vi "test_read-nmea-data2.vi"() -> ()   [LabVIEW 2019] (continued)
\n15:14:24.49\tF9P\t$GLGSV,2,1,08,69,10,031,37,70,70,037,25,71,54,207,25,72,05,210,,1*7E\n\t\n15:14:24.51\tF9P\t$GLGSV,2,2,08,77,01,325,,84,19,123,19,85,70,070,27,86,37,330,,1*7B\n\t\n15:14:24.53\tF9P\t$GLGSV,2,1,08,69,10,031,26,70,70,037,,71,54,207,16,72,05,210,,3*7B\n\t\n15:14:24.55\tF9P\t$GLGSV,2,2,08,77,01,325,,84,19,123,24,85,70,070,22,86,37,330,,3*72\n\t\n15:14:24.57\tF9P\t$GAGSV,2,1,08,02,08,296,11,04,67,115,26,09,33,193,24,11,72,001,24,7*7D\n\t\n15:14:24.59\tF9P\t$GAGSV,2,2,08,12,39,103,31,19,25,045,28,25,08,248,,36,27,309,18,7*74\n\t\n15:14:24.61\tF9P\t$GAGSV,2,1,08,02,08,296,,04,67,115,,09,33,193,,11,72,001,23,2*7D\n\t\n15:14:24.63\tF9P\t$GAGSV,2,2,08,12,39,103,27,19,25,045,,25,08,248,,36,27,309,,2*75\n\t\n15:14:24.65\tF9P\t$GBGSV,2,1,05,07,,,31,11,48,133,30,14,87,101,26,28,,,27,1*7A\n\t\n15:14:24.67\tF9P\t$GBGSV,2,2,05,33,62,220,24,1*41\n\t\n15:14:24.69\tF9P\t$GBGSV,1,1,03,11,48,133,31,14,87,101,28,33,62,220,,3*4C\n\t\n15:14:24.71\tF9P\t$GNGLL,3723.59802,N,12656.97828,E,061426.00,A,A*79\n\t\n15:14:24.73\tF9P\t\t\n15:14:24.75\tF9P\t\t\n15:14:24.77\tF9P\t\t\n15:14:24.79\tF9P\t\t\n15:14:24.81\tF9P\t\t\n15:14:24.83\tF9P\t\t\n15:14:24.85\tF9P\t\t\n15:14:24.87\tF9P\t\t\n15:14:24.89\tF9P\t\t\n15:14:24.91\tF9P\t\t\n15:14:24.93\tF9P\t\t\n15:14:24.95\tF9P\t\t\n15:14:24.97\tF9P\t\t\n15:14:24.99\tF9P\t\t\n15:14:25.01\tF9P\t\t\n15:14:25.03\tF9P\t\t\n15:14:25.05\tF9P\t\t\n15:14:25.07\tF9P\t\t\n15:14:25.09\tF9P\t\t\n15:14:25.11\tF9P\t\t\n15:14:25.13\tF9P\t\t\n15:14:25.15\tF9P\t\t\n15:14:25.17\tF9P\t\t\n15:14:25.19\tF9P\t\t\n15:14:25.21\tF9P\t\t\n15:14:25.23\tF9P\t$GNRMC,061427.00,A,3723.59868,N,12656.97826,E,2.049,344.09,25072\t\n15:14:25.25\tF9P\t0,,,A,V*00\n\t\n15:14:25.27\tF9P\t$GNVTG,344.09,T,,M,2.049,N,3.795,K,A*2E\n\t\n15:14:25.29\tF9P\t$GNGGA,061427.00,3723.59868,N,12656.97826,E,1,12,0.66,44.3,M,18.5,M,,*73\n\t\n15:14:25.31\tF9P\t$GNGSA,A,3,12,06,19,05,17,09,04,02,,,,,1.17,0.66,0.97,1*09\n\t\n15:14:25.33\tF9P\t$GNGSA,A,3,85,70,71,84,,,,,,,,,1.17,0.66,0.97,2*0B\n\t\n15:14:25.35\tF9P\t$GNGSA,A,3,36,19,11,04,09,12,,,,,,,1.17,0.66,0.97,3*09\n\t\n15:14:25.37\tF9P\t$GNGSA,A,3,14,11,33,,,,,,,,,,1.17,0.66,0.97,4*08\n\t\n15:14:25.39\tF9P\t$GPGSV,3,1,09,02,55,320,27,04,17,043,34,05,38,248,34,06,64,050,32,1*6C\n\t\n15:14:25.41\tF9P\t$GPGSV,3,2,09,09,44,073,31,12,23,276,30,17,32,154,27,19,51,157,30,1*6F\n\t\n15:14:25.43\tF9P\t$GPGSV,3,3,09,25,12,306,20,1*5E\n\t\n15:14:25.45\tF9P\t$GPGSV,3,1,09,02,55,320,,04,17,043,22,05,38,248,21,06,64,050,25,6*6B\n\t\n15:14:25.47\tF9P\t$GPGSV,3,2,09,09,44,073,25,12,23,276,14,17,32,154,23,19,51,157,,6*6C\n\t\n15:14:25.49\tF9P\t$GPGSV,3,3,09,25,12,306,,6*5B\n\t\n15:14:25.51\tF9P\t$GLGSV,2,1,08,69,10,031,35,70,70,037,24,71,54,207,25,72,05,210,,1*7D\n\t\n15:14:25.53\tF9P\t$GLGSV,2,2,08,77,01,325,,84,19,123,20,85,70,070,32,86,37,330,,1*75\n\t\n15:14:25.55\tF9P\t$GLGSV,2,1,08,69,10,031,26,70,70,037,,71,54,207,14,72,05,210,,3*79\n\t\n15:14:25.57\tF9P\t$GLGSV,2,2,08,77,01,325,,84,19,123,24,85,70,070,22,86,37,330,,3*72\n\t\n15:14:25.59\tF9P\t$GAGSV,2,1,08,02,08,296,08,04,67,115,25,09,33,193,24,11,72,001,25,7*77\n\t\n15:14:25.61\tF9P\t$GAGSV,2,2,08,12,39,103,27,19,25,045,29,25,08,248,,36,27,309,14,7*7E\n\t\n15:14:25.63\tF9P\t$GAGSV,2,1,08,02,08,296,,04,67,115,,09,33,193,,11,72,001,24,2*7A\n\t\n15:14:25.65\tF9P\t$GAGSV,2,2,08,12,39,103,25,19,25,045,,25,08,248,,36,27,309,,2*77\n\t\n15:14:25.67\tF9P\t$GBGSV,2,1,06,07,,,31,11,48,133,33,14,87,101,26,28,,,27,1*7A\n\t\n15:14:25.69\tF9P\t$GBGSV,2,2,06,33,62,220,26,34,,,43,1*40\n\t\n15:14:25.71\tF9P\t$GBGSV,1,1,03,11,48,133,30,14,87,101,,33,62,220,,3*47\n\t\n15:14:25.73\tF9P\t$GNGLL,3723.59868,N,12656.97826,E,061427.00,A,A*7A\n\t\n15:14:25.75\tF9P\t\t\n15:14:25.77\tF9P\t\t\n15:14:25.79\tF9P\t\t\n15:14:25.81\tF9P\t\t\n15:14:25.83\tF9P\t\t\n15:14:25.85\tF9P\t\t\n15:14:25.87\tF9P\t\t\n15:14:25.89\tF9P\t\t\n15:14:25.91\tF9P\t\t\n15:14:25.93\tF9P\t\t\n15:14:25.95\tF9P\t\t\n15:14:25.97\tF9P\t\t\n15:14:25.99\tF9P\t\t\n15:14:26.01\tF9P\t\t\n15:14:26.03\tF9P\t\t\n15:14:26.05\tF9P\t\t\n15:14:26.07\tF9P\t\t\n15:14:26.09\tF9P\t\t\n15:14:26.11\tF9P\t\t\n15:14:26.13\tF9P\t\t\n15:14:26.15\tF9P\t\t\n15:14:26.17\tF9P\t\t\n15:14:26.19\tF9P\t\t\n15:14:26.21\tF9P\t\t\n15:14:26.23\tF9P\t$GNRMC,061428.00,A,3723.59932,N,12656.97803,E,1.624,347.59,250720,,,A,V*0E\n\t\n15:14:26.25\tF9P\t$GNVTG,347.59,T,,M,1.624,N,3.007,K,A*2A\n\t\n15:14:26.27\tF9P\t$GNGGA,061428.00,3723.59932,N,12656.97803,E,1,12,0.71,44.3,M,18.5,M,,*73\n\t\n15:14:26.29\tF9P\t$GNGSA,A,3,12,06,19,05,17,09,04,02,,,,,1.23,0.71,1.01,1*06\n\t\n15:14:26.31\tF9P\t$GNGSA,A,3,85,70,71,84,,,,,,,,,1.23,0.71,1.01,2*04\n\t\n15:14:26.33\tF9P\t$GNGSA,A,3,36,19,11,04,09,12,,,,,,,1.23,0.71,1.01,3*06\n\t\n15:14:26.35\tF9P\t$GNGSA,A,3,14,11,33,,,,,,,,,,1.23,0.71,1.01,4*07\n\t\n15:14:26.37\tF9P\t$GPGSV,3,1,09,02,55,320,28,04,17,043,30,05,38,248,37,06,64,050,27,1*60\n\t\n15:14:26.39\tF9P\t$GPGSV,3,2,09,09,44,073,32,12,23,276,22,17,32,154,36,19,51,157,34,1*6B\n\t\n15:14:26.41\tF9P\t$GPGSV,3,3,09,25,12,306,21,1*5F\n\t\n15:14:26.43\tF9P\t$GPGSV,3,1,09,02,55,320,,04,17,043,22,05,38,248,20,06,64,050,26,6*69\n\t\n15:14:26.45\tF9P\t$GPGSV,3,2,09,09,44,073,26,12,23,276,15,17,32,154,23,19,51,157,,6*6E\n\t\n15:14:26.47\tF9P\t$GPGSV,3,3,09,25,12,306,,6*5B\n\t\n15:14:26.49\tF9P\t$GLGSV,2,1,08,69,10,031,28,70,70,037,23,71,54,207,24,72,05,210,,1*77\n\t\n15:14:26.51\tF9P\t$GLGSV,2,2,08,77,01,325,,84,19,123,20,85,70,070,33,86,37,330,,1*74\n\t\n15:14:26.53\tF9P\t$GLGSV,2,1,08,69,10,031,25,70,70,037,,71,54,207,15,72,05,210,,3*7B\n\t\n15:14:26.55\tF9P\t$GLGSV,2,2,08,77,01,325,,84,19,123,22,85,70,070,22,86,37,330,,3*74\n\t\n15:14:26.57\tF9P\t$GAGSV,2,1,08,02,08,296,10,04,67,115,31,09,33,193,24,11,72,001,25,7*7B\n\t\n15:14:26.59\tF9P\t$GAGSV,2,2,08,12,39,103,24,19,25,045,28,25,08,248,,36,27,309,12,7*7A\n\t\n15:14:26.61\tF9P\t$GAGSV,2,1,08,02,08,296,,04,67,115,,09,33,193,,11,72,001,,2*7C\n\t\n15:14:26.63\tF9P\t$GAGSV,2,2,08,12,39,103,23,19,25,045,,25,08,248,,36,27,309,,2*71\n\t\n15:14:26.65\tF9P\t$GBGSV,2,1,06,07,,,36,11,48,133,31,14,87,101,26,28,,,26,1*7E\n\t\n15:14:26.67\tF9P\t$GBGSV,2,2,06,33,62,220,42,34,,,40,1*41\n\t\n15:14:26.69\tF9P\t$GBGSV,1,1,03,11,48,133,,14,87,101,,33,62,220,,3*44\n\t\n15:14:26.71\tF9P\t$GNGLL,3723.59932,N,12656.97803,E,061428.00,A,A*7C\n\t\n15:14:26.73\tF9P\t\t\n15:14:26.75\tF9P\t\t\n15:14:26.77\tF9P\t\t\n15:14:26.79\tF9P\t\t\n15:14:26.81\tF9P\t\t\n15:14:26.83\tF9P\t\t\n15:14:26.85\tF9P\t\t\n15:14:26.87\tF9P\t\t\n15:14:26.89\tF9P\t\t\n15:14:26.91\tF9P\t\t\n15:14:26.93\tF9P\t\t\n15:14:26.95\tF9P\t\t\n15:14:26.97\tF9P\t\t\n15:14:26.99\tF9P\t\t\n15:14:27.01\tF9P\t\t\n15:14:27.03\tF9P\t\t\n15:14:27.05\tF9P\t\t\n15:14:27.07\tF9P\t\t\n15:14:27.09\tF9P\t\t\n15:14:27.11\tF9P\t\t\n15:14:27.13\tF9P\t\t\n15:14:27.15\tF9P\t\t\n15:14:27.17\tF9P\t\t\n15:14:27.19\tF9P\t\t\n15:14:27.21\tF9P\t\t\n15:14:27.23\tF9P\t\t\n15:14:27.25\tF9P\t$GNRMC,061429.00,A,3723.59979,N,12656.97808,E,1.116,354.33,250720,,,A,V*03\n\t\n15:14:27.27\tF9P\t$GNVTG,354.33,T,,M,1.116,N,2.066,K,A*24\n\t\n15:14:27.29\tF9P\t$GNGGA,061429.00,3723.59979,N,12656.97808,E,1,12,0.66,44.6,M,18.5,M,,*75\n\t\n15:14:27.31\tF9P\t$GNGSA,A,3,12,06,19,05,17,09,04,02,,,,,1.17,0.66,0.97,1*09\n\t\n15:14:27.33\tF9P\t$GNGSA,A,3,85,70,71,84,,,,,,,,,1.17,0.66,0.97,2*0B\n\t\n15:14:27.35\tF9P\t$GNGSA,A,3,36,19,11,04,09,12,,,,,,,1.17,0.66,0.97,3*09\n\t\n15:14:27.37\tF9P\t$GNGSA,A,3,14,11,33,,,,,,,,,,1.17,0.66,0.97,4*08\n\t\n15:14:27.39\tF9P\t$GPGSV,3,1,09,02,55,320,33,04,17,043,31,05,38,248,31,06,64,050,34,1*6F\n\t\n15:14:27.41\tF9P\t$GPGSV,3,2,09,09,44,073,31,12,23,276,22,17,32,154,31,19,51,157,37,1*6C\n\t\n15:14:27.43\tF9P\t$GPGSV,3,3,09,25,12,306,21,1*5F\n\t\n15:14:27.45\tF9P\t$GPGSV,3,1,09,02,55,320,,04,17,043,25,05,38,248,19,06,64,050,24,6*66\n\t\n15:14:27.47\tF9P\t$GPGSV,3,2,09,09,44,073,26,12,23,276,14,17,32,154,23,19,51,157,,6*6F\n\t\n15:14:27.49\tF9P\t$GPGSV,3,3,09,25,12,306,,6*5B\n\t\n15:14:27.51\tF9P\t$GLGSV,2,1,08,69,10,031,29,70,70,037,22,71,54,207,24,72,05,210,,1*77\n\t\n15:14:27.53\tF9P\t$GLGSV,2,2,08,77,01,325,,84,19,123,20,85,70,070,28,86,37,330,,1*7E\n\t\n15:14:27.55\tF9P\t$GLGSV,2,1,08,69,10,031,24,70,70,037,,71,54,207,16,72,05,210,,3*79\n\t\n15:14:27.57\tF9P\t$GLGSV,2,2,08,77,01,325,,84,19,123,22,85,70,070,24,86,37,330,,3*72\n\t\n15:14:27.59\tF9P\t$GAGSV,2,1,08,02,08,296,10,04,67,115,37,09,33,193,23,11,72,001,25,7*7A\n\t\n15:14:27.61\tF9P\t$GAGSV,2,2,08,12,39,103,25,19,25,045,28,25,08,248,,36,27,309,18,7*71\n\t\n15:14:27.63\tF9P\t$GAGSV,2,1,08,02,08,296,,04,67,115,,09,33,193,,11,72,001,,2*7C\n\t\n15:14:27.65\tF9P\t$GAGSV,2,2,08,12,39,103,22,19,25,045,,25,08,248,,36,27,309,,2*70\n\t\n15:14:27.67\tF9P\t$GBGSV,2,1,06,07,,,34,11,48,133,33,14,87,101,25,28,,,26,1*7D\n\t\n15:14:27.69\tF9P\t$GBGSV,2,2,06,33,62,220,37,34,,,42,1*41\n\t\n15:14:27.71\tF9P\t$GBGSV,1,1,03,11,48,133,29,14,87,101,,33,62,220,,3*4F\n\t\n15:14:27.73\tF9P\t$GNGLL,3723.59979,N,12656.97808,E,061429.00,A,A*79\n\t\n15:14:27.75\tF9P\t\t\n15:14:27.77\tF9P\t\t\n15:14:27.79\tF9P\t\t\n15:14:27.81\tF9P\t\t\n15:14:27.83\tF9P\t\t\n15:14:27.85\tF9P\t\t\n15:14:27.87\tF9P\t\t\n15:14:27.89\tF9P\t\t\n15:14:27.91\tF9P\t\t\n15:14:27.93\tF9P\t\t\n15:14:27.95\tF9P\t\t\n15:14:27.97\tF9P\t\t\n15:14:27.99\tF9P\t\t\n15:14:28.01\tF9P\t\t\n15:14:28.03\tF9P\t\t\n15:14:28.05\tF9P\t\t\n15:14:28.07\tF9P\t\t\n15:14:28.09\tF9P\t\t\n15:14:28.11\tF9P\t\t\n15:14:28.13\tF9P\t\t\n15:14:28.15\tF9P\t\t\n15:14:28.17\tF9P\t\t\n15:14:28.19\tF9P\t\t\n15:14:28.21\tF9P\t\t\n15:14:28.23\tF9P\t$GNRMC,061430.00,A,3723.60054,N,12656.97805,E,2.128,359.12,250720,,,A,V*0A\n\t\n15:14:28.25\tF9P\t$GNVTG,359.12,T,,M,2.128,N,3.941,K,A*29\n\t\n15:14:28.27\tF9P\t$GNGGA,061430.00,3723.60054,N,12656.97805,E,1,12,0.66,44.5,M,18.5,M,,*7F\n\t\n15:14:28.29\tF9P\t$GNGSA,A,3,12,06,19,05,17,09,04,02,,,,,1.17,0.66,0.97,1*09\n\t\n15:14:28.31\tF9P\t$GNGSA,A,3,85,70,71,84,,,,,,,,,1.17,0.66,0.97,2*0B\n\t\n15:14:28.33\tF9P\t$GNGSA,A,3,36,19,11,04,09,12,,,,,,,1.17,0.66,0.97,3*09\n\t\n15:14:28.35\tF9P\t$GNGSA,A,3,14,11,33,,,,,,,,,,1.17,0.66,0.97,4*08\n\t\n15:14:28.37\tF9P\t$GPGSV,3,1,09,02,55,320,23,04,17,043,34,05,38,248,25,06,64,050,25,1*6E\n\t\n15:14:28.39\tF9P\t$GPGSV,3,2,09,09,44,073,30,12,23,276,23,17,32,154,41,19,51,157,34,1*68\n\t\n15:14:28.41\tF9P\t$GPGSV,3,3,09,25,12,306,20,1*5E\n\t\n15:14:28.43\tF9P\t$GPGSV,3,1,09,02,55,320,,04,17,043,24,05,38,248,18,06,64,050,23,6*61\n\t\n15:14:28.45\tF9P\t$GPGSV,3,2,09,09,44,073,25,12,23,276,13,17,32,154,22,19,51,157,,6*6A\n\t\n15:14:28.47\tF9P\t$GPGSV,3,3,09,25,12,306,,6*5B\n\t\n15:14:28.49\tF9P\t$GLGSV,2,1,08,69,10,031,34,70,70,037,22,71,54,207,23,72,05,210,,1*7C\n\t\n15:14:28.51\tF9P\t$GLGSV,2,2,08,77,01,325,,84,19,123,19,85,70,070,34,86,37,330,,1*79\n\t\n15:14:28.53\tF9P\t$GLGSV,2,1,08,69,10,031,22,70,70,037,,71,54,207,15,72,05,210,,3*7C\n\t\n15:14:28.55\tF9P\t$GLGSV,2,2,08,77,01,325,,84,19,123,22,85,70,070,24,86,37,330,,3*72\n\t\n15:14:28.57\tF9P\t$GAGSV,2,1,08,02,08,296,08,04,67,115,31,09,33,193,23,11,72,001,24,7*74\n\t\n15:14:28.59\tF9P\t$GAGSV,2,2,08,12,39,103,31,19,25,045,28,25,08,248,,36,27,309,18,7*74\n\t\n15:14:28.61\tF9P\t$GAGSV,2,1,08,02,08,296,,04,67,115,,09,33,193,,11,72,001,,2*7C\n\t\n15:14:28.63\tF9P\t$GAGSV,2,2,08,12,39,103,23,19,25,045,,25,08,248,,36,27,309,,2*71\n\t\n15:14:28.65\tF9P\t$GBGSV,2,1,06,07,,,26,11,48,133,35,14,87,101,25,28,,,25,1*7B\n\t\n15:14:28.67\tF9P\t$GBGSV,2,2,06,33,62,220,35,34,,,41,1*40\n\t\n15:14:28.69\tF9P\t$GBGSV,1,1,03,11,48,133,33,14,87,101,,33,62,220,,3*44\n\t\n15:14:28.71\tF9P\t$GNGLL,3723.60054,N,12656.97805,E,061430.00,A,A*70\n\t\n15:14:28.73\tF9P\t\t\n15:14:28.75\tF9P\t\t\n15:14:28.77\tF9P\t\t\n15:14:28.79\tF9P\t\t\n15:14:28.81\tF9P\t\t\n15:14:28.83\tF9P\t\t\n15:14:28.85\tF9P\t\t\n15:14:28.87\tF9P\t\t\n15:14:28.89\tF9P\t\t\n15:14:28.91\tF9P\t\t\n15:14:28.93\tF9P\t\t\n15:14:28.95\tF9P\t\t\n15:14:28.97\tF9P\t\t\n15:14:28.99\tF9P\t\t\n15:14:29.01\tF9P\t\t\n15:14:29.03\tF9P\t\t\n15:14:29.05\tF9P\t\t\n15:14:29.07\tF9P\t\t\n15:14:29.09\tF9P\t\t\n15:14:29.11\tF9P\t\t\n15:14:29.13\tF9P\t\t\n15:14:29.15\tF9P\t\t\n15:14:29.17\tF9P\t\t\n15:14:29.19\tF9P\t\t\n15:14:29.21\tF9P\t\t\n15:14:29.23\tF9P\t\t\n15:14:29.25\tF9P\t$GNRMC,061431.00,A,3723.60124,N,12656.97773,E,1.697,350.54,250720,,,A,V*08\n\t\n15:14:29.27\tF9P\t$GNVTG,350.54,T,,M,1.697,N,3.142,K,A*29\n\t\n15:14:29.29\tF9P\t$GNGGA,061431.00,3723.60124,N,12656.97773,E,1,12,0.66,44.5,M,18.5,M,,*76\n\t\n15:14:29.31\tF9P\t$GNGSA,A,3,12,06,19,05,17,09,04,02,,,,,1.17,0.66,0.97,1*09\n\t\n15:14:29.33\tF9P\t$GNGSA,A,3,85,70,71,84,,,,,,,,,1.17,0.66,0.97,2*0B\n\t\n15:14:29.35\tF9P\t$GNGSA,A,3,36,19,11,04,09,12,,,,,,,1.17,0.66,0.97,3*09\n\t\n15:14:29.37\tF9P\t$GNGSA,A,3,14,11,33,,,,,,,,,,1.17,0.66,0.97,4*08\n\t\n15:14:29.39\tF9P\t$GPGSV,3,1,09,02,55,320,25,04,17,043,30,05,38,248,31,06,64,050,24,1*68\n\t\n15:14:29.41\tF9P\t$GPGSV,3,2,09,09,44,073,33,12,23,276,22,17,32,154,37,19,51,157,33,1*6C\n\t\n15:14:29.43\tF9P\t$GPGSV,3,3,09,25,12,306,21,1*5F\n\t\n15:14:29.45\tF9P\t$GPGSV,3,1,09,02,55,320,,04,17,043,30,05,38,248,17,06,64,050,24,6*6C\n\t\n15:14:29.47\tF9P\t$GPGSV,3,2,09,09,44,073,25,12,23,276,10,17,32,154,22,19,51,157,,6*69\n\t\n15:14:29.49\tF9P\t$GPGSV,3,3,09,25,12,306,,6*5B\n\t\n15:14:29.51\tF9P\t$GLGSV,2,1,08,69,10,031,32,70,70,037,23,71,54,207,25,72,05,210,,1*7D\n\t\n15:14:29.53\tF9P\t$GLGSV,2,2,08,77,01,325,,84,19,123,20,85,70,070,29,86,37,330,,1*7F\n\t\n15:14:29.55\tF9P\t$GLGSV,2,1,08,69,10,031,22,70,70,037,,71,54,207,15,72,05,210,,3*7C\n\t\n15:14:29.57\tF9P\t$GLGSV,2,2,08,77,01,325,,84,19,123,23,85,70,070,24,86,37,330,,3*73\n\t\n15:14:29.59\tF9P\t$GAGSV,2,1,08,02,08,296,10,04,67,115,34,09,33,193,24,11,72,001,25,7*7E\n\t\n15:14:29.61\tF9P\t$GAGSV,2,2,08,12,39,103,31,19,25,045,27,25,08,248,,36,27,309,20,7*70\n\t\n15:14:29.63\tF9P\t$GAGSV,2,1,08,02,08,296,,04,67,115,,09,33,193,,11,72,001,,2*7C\n\t\n15:14:29.65\tF9P\t$GAGSV,2,2,08,12,39,103,24,19,25,045,,25,08,248,,36,27,309,,2*76\n\t\n15:14:29.67\tF9P\t$GBGSV,2,1,06,07,,,32,11,48,133,31,14,87,101,24,28,,,26,1*78\n\t\n15:14:29.69\tF9P\t$GBGSV,2,2,06,33,62,220,35,34,,,42,1*43\n\t\n15:14:29.71\tF9P\t$GBGSV,1,1,03,11,48,133,27,14,87,101,,33,62,220,,3*41\n\t\n15:14:29.73\tF9P\t$GNGLL,3723.60124,N,12656.97773,E,061431.00,A,A*79\n\t\n15:14:29.75\tF9P\t\t\n15:14:29.77\tF9P\t\t\n15:14:29.79\tF9P\t\t\n15:14:29.81\tF9P\t\t\n15:14:29.83\tF9P\t\t\n15:14:29.85\tF9P\t\t\n15:14:29.87\tF9P\t\t\n15:14:29.89\tF9P\t\t\n15:14:29.91\tF9P\t\t\n15:14:29.93\tF9P\t\t\n15:14:29.95\tF9P\t\t\n15:14:29.97\tF9P\t\t\n15:14:29.99\tF9P\t\t\n15:14:30.01\tF9P\t\t\n15:14:30.03\tF9P\t\t\n15:14:30.05\tF9P\t\t\n15:14:30.07\tF9P\t\t\n15:14:30.09\tF9P\t\t\n15:14:30.11\tF9P\t\t\n15:14:30.13\tF9P\t\t\n15:14:30.15\tF9P\t\t\n15:14:30.17\tF9P\t\t\n15:14:30.19\tF9P\t\t\n15:14:30.21\tF9P\t\t\n15:14:30.23\tF9P\t$GNRMC,061432.00,A,3723.60177,N,12656.97725,E,1.531,335.45,250720,,,A,V*02\n\t\n15:14:30.25\tF9P\t$GNVTG,335.45,T,,M,1.531,N,2.836,K,A*2E\n\t\n15:14:30.27\tF9P\t$GNGGA,061432.00,3723.60177,N,12656.97725,E,1,12,0.69,44.6,M,18.5,M,,*7C\n\t\n15:14:30.29\tF9P\t$GNGSA,A,3,12,06,19,05,17,09,04,02,,,,,1.22,0.69,1.00,1*0F\n\t\n15:14:30.31\tF9P\t$GNGSA,A,3,85,70,71,84,,,,,,,,,1.22,0.69,1.00,2*0D\n\t\n15:14:30.33\tF9P\t$GNGSA,A,3,36,19,11,04,09,12,,,,,,,1.22,0.69,1.00,3*0F\n\t\n15:14:30.35\tF9P\t$GNGSA,A,3,14,11,33,,,,,,,,,,1.22,0.69,1.00,4*0E\n\t\n15:14:30.37\tF9P\t$GPGSV,3,1,09,02,55,320,25,04,17,043,33,05,38,248,37,06,64,050,31,1*69\n\t\n15:14:30.39\tF9P\t$GPGSV,3,2,09,09,44,073,29,12,23,276,22,17,32,154,41,19,51,157,37,1*62\n\t\n15:14:30.41\tF9P\t$GPGSV,3,3,09,25,12,306,22,1*5C\n\t\n15:14:30.43\tF9P\t$GPGSV,3,1,09,02,55,320,,04,17,043,31,05,38,248,17,06,64,050,30,6*68\n\t\n15:14:30.45\tF9P\t$GPGSV,3,2,09,09,44,073,25,12,23,276,12,17,32,154,22,19,51,157,,6*6B\n\t\n15:14:30.47\tF9P\t$GPGSV,3,3,09,25,12,306,,6*5B\n\t\n15:14:30.49\tF9P\t$GLGSV,2,1,08,69,10,031,28,70,70,037,23,71,54,207,26,72,05,210,,1*75\n\t\n15:14:30.51\tF9P\t$GLGSV,2,2,08,77,01,324,,84,19,123,20,85,70,070,29,86,37,330,,1*7E\n\t\n15:14:30.53\tF9P\t$GLGSV,2,1,08,69,10,031,22,70,70,037,,71,54,207,17,72,05,210,,3*7E\n\t\n15:14:30.55\tF9P\t$GLGSV,2,2,08,77,01,324,,84,19,123,23,85,70,070,23,86,37,330,,3*75\n\t\n15:14:30.57\tF9P\t$GAGSV,2,1,08,02,08,296,10,04,67,115,25,09,33,193,24,11,72,001,25,7*7E\n\t\n15:14:30.59\tF9P\t$GAGSV,2,2,08,12,39,103,30,19,25,045,31,25,08,248,,36,27,309,20,7*76\n\t\n15:14:30.61\tF9P\t$GAGSV,2,1,08,02,08,296,,04,67,115,,09,33,193,,11,72,001,,2*7C\n\t\n15:14:30.63\tF9P\t$GAGSV,2,2,08,12,39,103,,19,25,045,,25,08,248,,36,27,309,,2*70\n\t\n15:14:30.65\tF9P\t$GBGSV,2,1,06,07,,,26,11,48,133,34,14,87,101,26,28,,,25,1*79\n\t\n15:14:30.67\tF9P\t$GBGSV,2,2,06,33,62,220,37,34,,,40,1*43\n\t\n15:14:30.69\tF9P\t$GBGSV,1,1,03,11,48,133,33,14,87,101,,33,62,220,,3*44\n\t\n15:14:30.71\tF9P\t$GNGLL,3723.60177,N,12656.97725,E,061432.00,A,A*7F\n\t\n15:14:30.73\tF9P\t\t\n15:14:30.75\tF9P\t\t\n15:14:30.77\tF9P\t\t\n15:14:30.79\tF9P\t\t\n15:14:30.81\tF9P\t\t\n15:14:30.83\tF9P\t\t\n15:14:30.85\tF9P\t\t\n15:14:30.87\tF9P\t\t\n15:14:30.89\tF9P\t\t\n15:14:30.91\tF9P\t\t\n15:14:30.93\tF9P\t\t\n15:14:30.95\tF9P\t\t\n15:14:30.97\tF9P\t\t\n15:14:30.99\tF9P\t\t\n15:14:31.01\tF9P\t\t\n15:14:31.03\tF9P\t\t\n15:14:31.05\tF9P\t\t\n15:14:31.07\tF9P\t\t\n15:14:31.09\tF9P\t\t\n15:14:31.11\tF9P\t\t\n15:14:31.13\tF9P\t\t\n15:14:31.15\tF9P\t\t\n15:14:31.17\tF9P\t\t\n15:14:31.19\tF9P\t\t\n15:14:31.21\tF9P\t\t\n15:14:31.23\tF9P\t$GNRMC,061433.00,A,3723.60224,N,12656.97709,E,1.157,339.88,250720,,,A,V*01\n\t\n15:14:31.25\tF9P\t$GNVTG,339.88,T,,M,1.157,N,2.143,K,A*2C\n\t\n15:14:31.27\tF9P\t$GNGGA,061433.00,3723.60224,N,12656.97709,E,1,12,0.66,44.6,M,18.5,M,,*79\n\t\n15:14:31.29\tF9P\t$GNGSA,A,3,12,06,19,05,17,09,04,02,,,,,1.17,0.66,0.97,1*09\n\t\n15:14:31.31\tF9P\t$GNGSA,A,3,85,70,71,84,,,,,,,,,1.17,0.66,0.97,2*0B\n\t\n15:14:31.33\tF9P\t$GNGSA,A,3,36,19,11,04,09,12,,,,,,,1.17,0.66,0.97,3*09\n\t\n15:14:31.35\tF9P\t$GNGSA,A,3,14,11,33,,,,,,,,,,1.17,0.66,0.97,4*08\n\t\n15:14:31.37\tF9P\t$GPGSV,3,1,09,02,55,320,27,04,17,043,35,05,38,248,28,06,64,050,26,1*65\n\t\n15:14:31.39\tF9P\t$GPGSV,3,2,09,09,44,073,37,12,23,276,22,17,32,154,32,19,51,157,35,1*6B\n\t\n15:14:31.41\tF9P\t$GPGSV,3,3,09,25,12,306,22,1*5C\n\t\n15:14:31.43\tF9P\t$GPGSV,3,1,09,02,55,320,,04,17,043,26,05,38,248,17,06,64,050,25,6*6A\n\t\n15:14:31.45\tF9P\t$GPGSV,3,2,09,09,44,073,26,12,23,276,13,17,32,154,21,19,51,157,,6*6A\n\t\n15:14:31.47\tF9P\t$GPGSV,3,3,09,25,12,306,,6*5B\n\t\n15:14:31.49\tF9P\t$GLGSV,2,1,08,69,10,031,32,70,70,037,22,71,54,207,32,72,05,210,,1*7A\n\t\n15:14:31.51\tF9P\t$GLGSV,2,2,08,77,01,324,,84,19,123,20,85,70,070,32,86,37,330,,1*74\n\t\n15:14:31.53\tF9P\t$GLGSV,2,1,08,69,10,031,22,70,70,037,,71,54,207,21,72,05,210,,3*7B\n\t\n15:14:31.55\tF9P\t$GLGSV,2,2,08,77,01,324,,84,19,123,22,85,70,070,23,86,37,330,,3*74\n\t\n15:14:31.57\tF9P\t$GAGSV,2,1,08,02,08,296,09,04,67,115,30,09,33,193,25,11,72,001,25,7*73\n\t\n15:14:31.59\tF9P\t$GAGSV,2,2,08,12,39,103,31,19,25,045,25,25,08,248,,36,27,309,20,7*72\n\t\n15:14:31.61\tF9P\t$GAGSV,2,1,08,02,08,296,,04,67,115,,09,33,193,,11,72,001,,2*7C\n\t\n15:14:31.63\tF9P\t$GAGSV,2,2,08,12,39,103,,19,25,045,,25,08,248,,36,27,309,,2*70\n\t\n15:14:31.65\tF9P\t$GBGSV,2,1,06,07,,,28,11,48,133,41,14,87,101,26,28,,,30,1*71\n\t\n15:14:31.67\tF9P\t$GBGSV,2,2,06,33,62,220,30,34,,,43,1*47\n\t\n15:14:31.69\tF9P\t$GBGSV,1,1,03,11,48,133,30,14,87,101,27,33,62,220,,3*42\n\t\n15:14:31.71\tF9P\t$GNGLL,3723.60224,N,12656.97709,E,061433.00,A,A*75\n\t\n15:14:31.73\tF9P\t\t\n15:14:31.75\tF9P\t\t\n15:14:31.77\tF9P\t\t\n15:14:31.79\tF9P\t\t\n15:14:31.81\tF9P\t\t\n15:14:31.83\tF9P\t\t\n15:14:31.85\tF9P\t\t\n15:14:31.87\tF9P\t\t\n15:14:31.89\tF9P\t\t\n15:14:31.91\tF9P\t\t\n15:14:31.93\tF9P\t\t\n15:14:31.95\tF9P\t\t\n15:14:31.97\tF9P\t\t\n15:14:31.99\tF9P\t\t\n15:14:32.01\tF9P\t\t\n15:14:32.03\tF9P\t\t\n15:14:32.05\tF9P\t\t\n15:14:32.07\tF9P\t\t\n15:14:32.09\tF9P\t\t\n15:14:32.11\tF9P\t\t\n15:14:32.13\tF9P\t\t\n15:14:32.15\tF9P\t\t\n15:14:32.17\tF9P\t\t\n15:14:32.19\tF9P\t\t\n15:14:32.21\tF9P\t\t\n15:14:32.23\tF9P\t$GNRMC,061434.00,A,3723.60300,N,12656.97670,E,2.413,340.67,250720,,,A,V*07\n\t\n15:14:32.25\tF9P\t$GNVTG,340.67,T,,M,2.413,N
